vi "init.vi"(8 "error in (no error)":errorcluster, 11 "Protocol_a in":refnum<class "Protocol_a.lvclass">) -> (0 "error out":errorcluster, 3 "Protocol_a out":refnum<class "Protocol_a.lvclass">)   [LabVIEW 2011, in "Protocol_A.lvclass"]
uses:
  Protocol_a.lvclass
  protocol_Generic/Protocol_Generic.lvclass
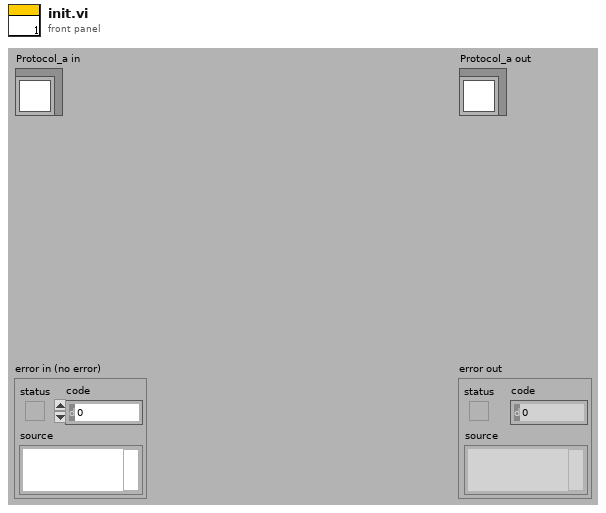
[diagram p1: front panel]
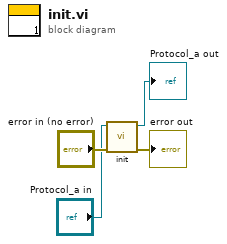
[diagram p0: block diagram]
diagram:
  n1 = call-parent "init.vi"("error in (no error)"="error in (no error)", "Protocol_Generic in"="Protocol_a in") -> ("error out"=→"error out":errorcluster, "Protocol_Generic out"=→"Protocol_a out":refnum<class "Protocol_a.lvclass">)  [unwired: 8 in]
